vi "Intake Wheels Logic.vi"(11 "Intake Seen":bool) -> (1 "Done":bool, 2 "Carrage Output":dbl=-1.0, 3 "Intake Output":dbl=1.0)   [LabVIEW 2017]
uses:
  Robot Global Data.vi
panel:
  in  "Time Target (s)":dbl=0.25 format="%#_13g"
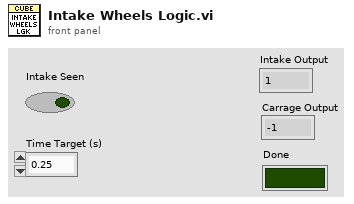
[diagram p1: front panel]
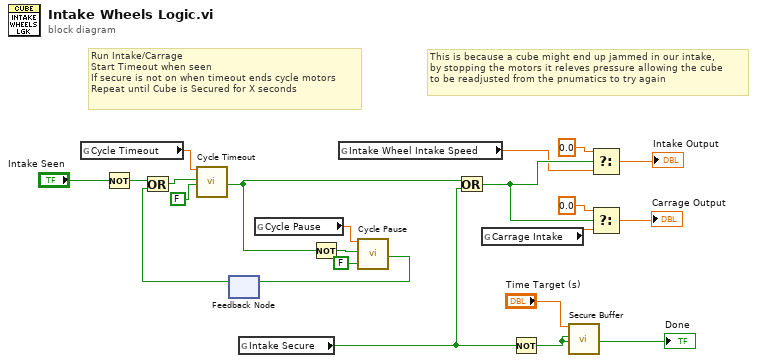
[diagram p0: block diagram]
diagram:
  # "This is because a cube might end up jammed in our intake,\nby stopping the motors it releves pressure allowing the cube\nto be readjusted from the pnumatics to try again"
  # "Run Intake/Carrage\nStart Timeout when seen\nIf secure is not on when timeout ends cycle motors\nRepeat until Cube is Secured for X seconds"
  n1 = global read "Robot Global Data.vi" "Cycle Timeout"() -> (w18:dbl)
  n2 = Not(x="Intake Seen") -> (.not. x?=w19:bool)
  n3 = feedback #1() -> (w13:bool)  [unwired: 1 in]
  n4 = Or(x=w19, y=w13) -> (x .or. y?=w15:bool)
  n5 = call "Cycle Timeout"("Time Target (s)"=w18, "Reset"=w15, "Auto Reset"=FALSE) -> ("Time has Elapsed"=w7:bool)  [unwired: 9 in, 7 out]
  n6 = global read "Robot Global Data.vi" "Intake Secure"() -> (w9:bool)
  n7 = global read "Robot Global Data.vi" "Cycle Pause"() -> (w17:dbl)
  n8 = Not(x=w7) -> (.not. x?=w16:bool)
  n9 = global read "Robot Global Data.vi" "Intake Wheel Intake Speed"() -> (w1:dbl)
  n10 = call "Cycle Pause"("Time Target (s)"=w17, "Reset"=w16, "Auto Reset"=FALSE) -> ("Time has Elapsed"=w14:bool)  [unwired: 9 in, 7 out]
  n11 = feedback-in #1(w14) -> ()
  n12 = Or(x=w7, y=w9) -> (x .or. y?=w12:bool)
  n13 = global read "Robot Global Data.vi" "Carrage Intake"() -> (w4:dbl)
  n14 = Not(x=w9) -> (.not. x?=w10:bool)
  n15 = call "Secure Buffer"("Time Target (s)"="Time Target (s)", "Reset"=w10, "Auto Reset"=w10) -> ("Time has Elapsed"=→"Done":bool)  [unwired: 9 in, 7 out]
  n16 = Select(t=0.0, s=w12, f=w1) -> (s? t:f=→"Intake Output":dbl)
  n17 = Select(t=0.0, s=w12, f=w4) -> (s? t:f=→"Carrage Output":dbl)
